vi "数据库读取.vi"(8 "error in (no error)":errorcluster caption="错误输入（无错误）", 11 "列表选择":T1(ring)) -> (0 "error out":errorcluster caption="错误输出", 1 "远程数据":string[][](table), 2 "本地数据":string[][](table), 3 "有未发送数据":bool)   [LabVIEW 2016, in "数据传输系统-03.lvlib"]
uses:
  <vilib>/Utility/sysdir.llb/System Directory Type.ctl
  <vilib>/addons/database/Connection.llb/DB Tools Open Connec (String).vi
  <vilib>/addons/database/_DB Variant To Data/Database Variant To Data.xnode
  <vilib>/addons/database/NI_Database_API.lvlib
panel:
  out "远程数据 2":string[][](table)
  out "x-y":i32[](array[numeric])
  out "大小 2":i32[](array[numeric])
  out "大小":i32[](array[numeric])
  out "待发送数据量":i32
  out "已发送数据量":i32
  out "error out 2":errorcluster caption="错误输出"
  in  "error in (no error) 2":errorcluster caption="错误输入（无错误）"
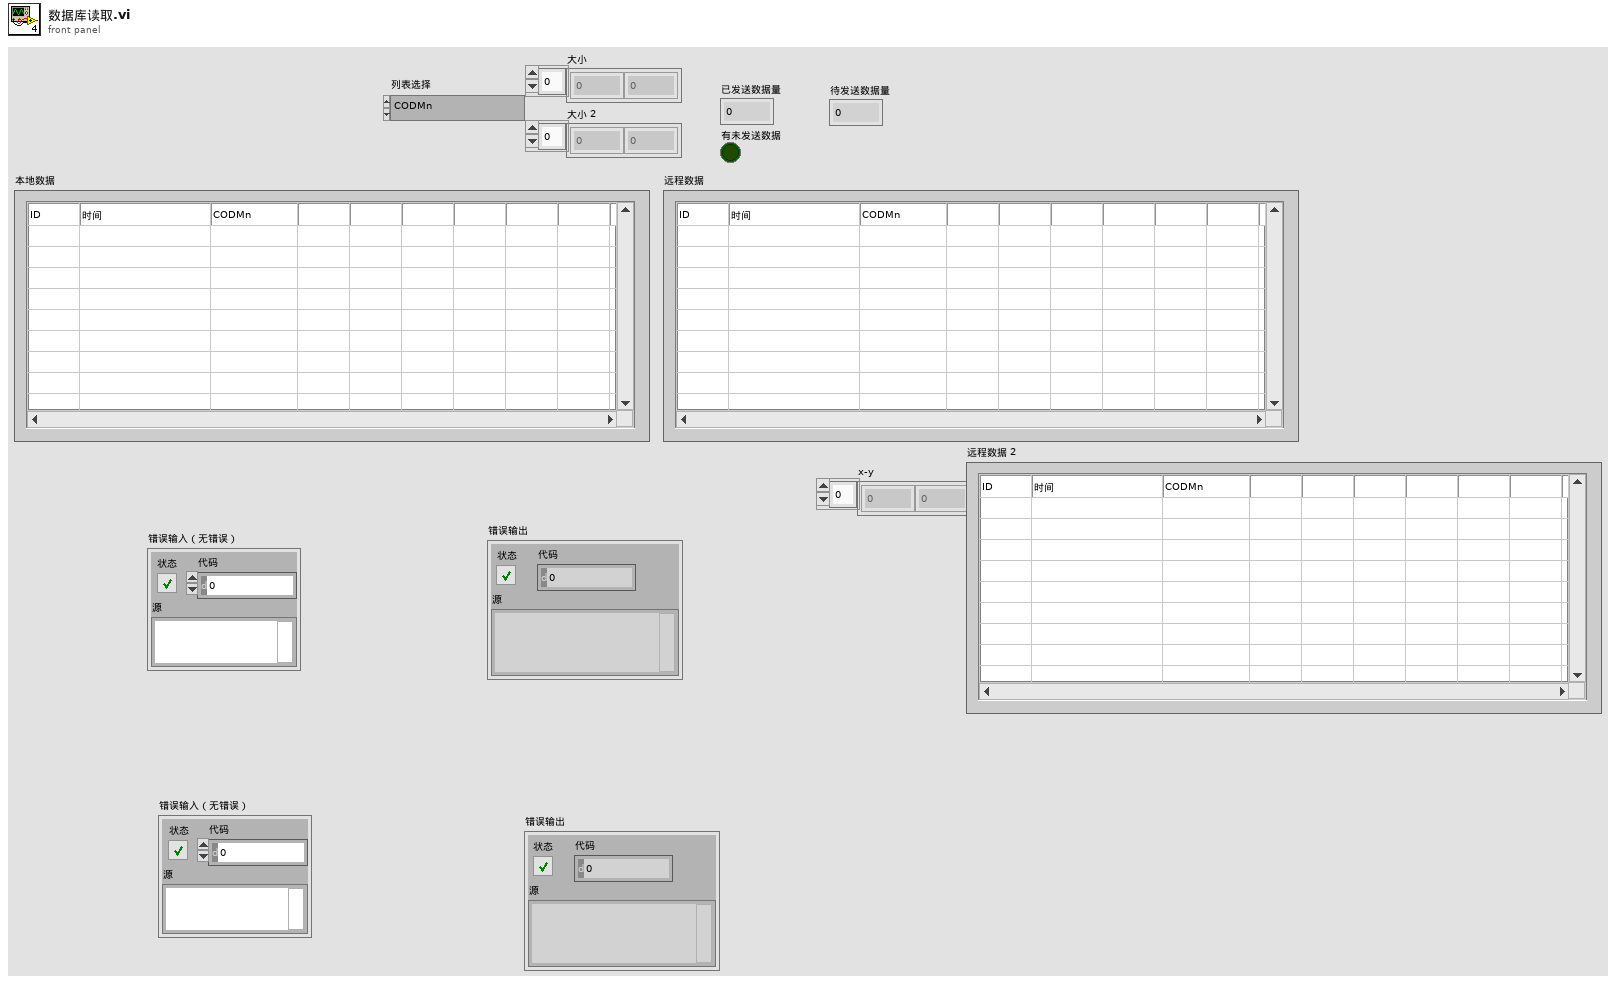
[diagram p1: front panel]
types:
  T1 = enum16{"CODMn", "CODMn空白核查", "CODMn标样核查", "氨氮", "氨氮空白核查", "氨氮标样核查", "多参数", "多参标样核查", "总磷", "总磷空白核查", "总磷标样核查", "总氮", "总氮空白核查", "总氮标样核查"}
  T2 = typedef "System Directory Type.ctl" = i32
  T3 = typedef "NI_Database_API.lvlib/Conn ObjectReference.ctl" = refnum<k1>
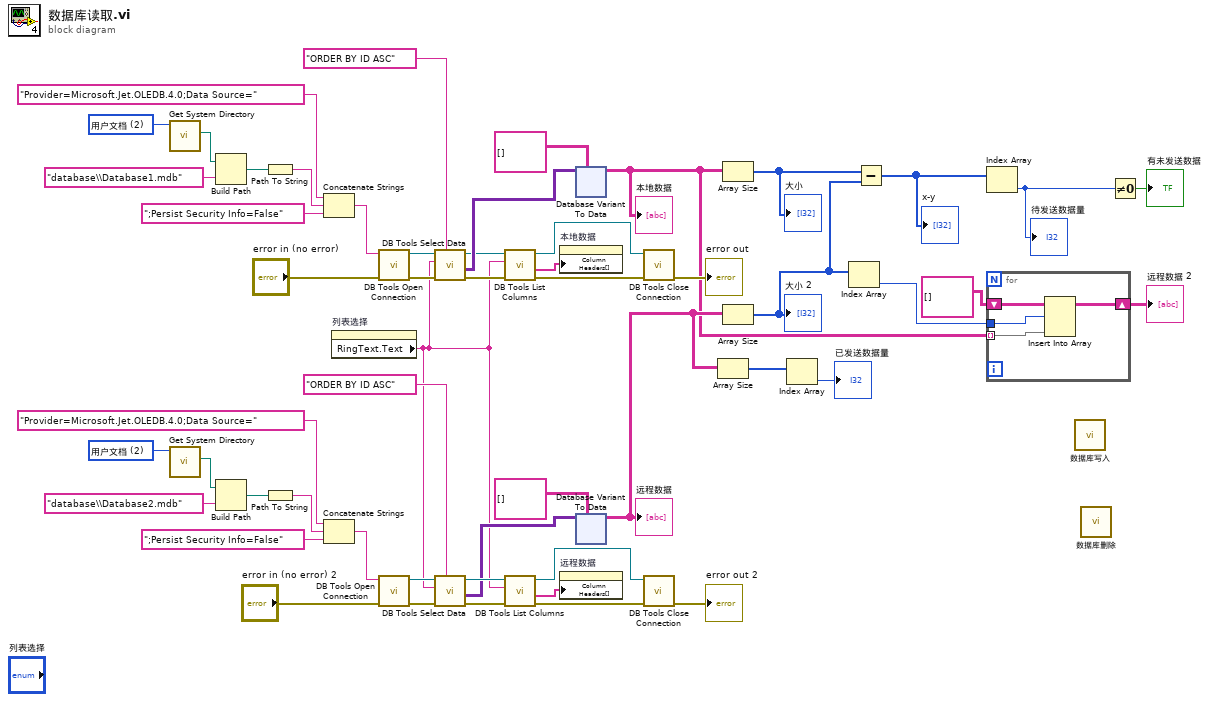
[diagram p0: block diagram]
diagram:
  w26 = T2 2 items=["用户目录"=0, "用户桌面"=1, "用户文档"=2, "用户应用程序数据"=3, "用户设置"=4, "用户临时目录"=5, "公共文档"=6, "公共应用程序数据"=7, "公共设置"=8, "公共缓存"=13, "系统核心库"=9, "系统安装库"=10, "应用程序文件"=11, "启动盘根目录"=12] ("system directory type")
  w41 = T2 2 items=["用户目录"=0, "用户桌面"=1, "用户文档"=2, "用户应用程序数据"=3, "用户设置"=4, "用户临时目录"=5, "公共文档"=6, "公共应用程序数据"=7, "公共设置"=8, "公共缓存"=13, "系统核心库"=9, "系统安装库"=10, "应用程序文件"=11, "启动盘根目录"=12] ("system directory type")
  n1 = call <vilib>:"Get System Directory.vi"("system directory type"=w41) -> ("system directory"=w39:path)  [unwired: 10 in]
  n2 = call <vilib>:"Get System Directory.vi"("system directory type"=w26) -> ("system directory"=w28:path)  [unwired: 10 in]
  n3 = Build Path(base path=w39, name or relative path="database\\Database1.mdb" ("condition")) -> (appended path=w37:path)
  n4 = Build Path(base path=w28, name or relative path="database\\Database2.mdb" ("condition")) -> (appended path=w30:path)
  n5 = Path To String(path=w37) -> (string=w36:string)
  n6 = Path To String(path=w30) -> (string=w31:string)
  n7 = Concatenate Strings("Provider=Microsoft.Jet.OLEDB.4.0;Data Source=" ("condition"), w36, ";Persist Security Info=False" ("condition")) -> (w34:string)
  n8 = Concatenate Strings("Provider=Microsoft.Jet.OLEDB.4.0;Data Source=" ("condition"), w31, ";Persist Security Info=False" ("condition")) -> (w33:string)
  n9 = property on="列表选择" class="Enum (严格)"() -> ("RingText.Text"=w11:string)  [unwired: 2 in, 2 out]
  n10 = call-poly <vilib>:"DB Tools Open Connection.vi"("error in (no error)"="error in (no error)", "connection information"=w34) -> ("error out"=w52:errorcluster, "connection reference"=w53:T3)  [unwired: 6 in]
  n11 = call-poly <vilib>:"DB Tools Open Connection.vi"("error in (no error)"="error in (no error) 2", "connection information"=w33) -> ("error out"=w21:errorcluster, "connection reference"=w20:T3)  [unwired: 6 in]
  n12 = call <vilib>:"DB Tools Select Data.vi"("condition"="ORDER BY ID ASC", "error in (no error)"=w52, "table"=w11, "connection reference"=w53) -> ("error out"=w47:errorcluster, "data"=w51:variant[][], "connection reference out"=w48:T3)  [unwired: 2 in]
  n13 = call <vilib>:"DB Tools Select Data.vi"("condition"="ORDER BY ID ASC", "error in (no error)"=w21, "table"=w11, "connection reference"=w20) -> ("error out"=w24:errorcluster, "data"=w18:variant[][], "connection reference out"=w23:T3)  [unwired: 2 in]
  n14 = call <vilib>:"DB Tools List Columns.vi"("error in (no error)"=w47, "table"=w11, "connection reference"=w48) -> ("error out"=w46:errorcluster, "columns"=w43:string[], "connection reference out"=w45:T3)  [unwired: 1 in, 1 out]
  n15 = call <vilib>:"DB Tools List Columns.vi"("error in (no error)"=w24, "table"=w11, "connection reference"=w23) -> ("error out"=w14:errorcluster, "columns"=w17:string[], "connection reference out"=w15:T3)  [unwired: 1 in, 1 out]
  n16 = property on="本地数据" class="Tbl (严格)"("Column Headers[]"=w43) -> ()  [unwired: 2 in, 2 out]
  n17 = property on="远程数据" class="Tbl (严格)"("Column Headers[]"=w17) -> ()  [unwired: 2 in, 2 out]
  n18 = xnode "Database Variant To Data"("database variant"=w51, "type"=string[][] []) -> ("data"=w3:string[][])  [unwired: 1 in, 1 out]
  "本地数据" <- w3
  n19 = xnode "Database Variant To Data"("database variant"=w18, "type"=string[][] []) -> ("data"=w10:string[][])  [unwired: 1 in, 1 out]
  "远程数据" <- w10
  n20 = call <vilib>:"DB Tools Close Connection.vi"("error in (no error)"=w46, "connection reference"=w45) -> ("error out"=→"error out":errorcluster)  [unwired: 5 in]
  n21 = call <vilib>:"DB Tools Close Connection.vi"("error in (no error)"=w14, "connection reference"=w15) -> ("error out"=→"error out 2":errorcluster)  [unwired: 5 in]
  n22 = Array Size(array=w10) -> (size(s)=w13:i32[])
  n23 = Array Size(array=w3) -> (size(s)=w6:i32[])
  "大小" <- w6
  n24 = Array Size(array=w10) -> (size(s)=w5:i32[])
  "大小 2" <- w5
  n25 = Index Array(array=w13) -> (element=→"已发送数据量":i32)  [unwired: 1 in]
  n26 = Index Array(array=w5) -> (element=w4:i32)  [unwired: 1 in]
  n27 = Subtract(x=w6, y=w5) -> (x-y=w9:i32[])
  "x-y" <- w9
  n28 = Index Array(array=w9) -> (element=w7:i32)  [unwired: 1 in]
  "待发送数据量" <- w7
  n29 = for {
    tunnel: w3 -> [w55] mode=indexing
    tunnel: w4 -> [w56]
    shift-right: [w54] -> w2
    shift-left: string[][] [] -> [w57]
    n30 = Insert Into Array(array=w57, index (row)=w56, new element=w55) -> (w54:string[][])  [unwired: 1 in]
  }
  "远程数据 2" <- w2
  n31 = call "数据库写入.vi"() -> ()  [unwired: 18 in, 2 out]
  n32 = call "数据库删除.vi"() -> ()  [unwired: 9 in, 3 out]
  n33 = Not Equal To 0?(x=w7) -> (x != 0?=→"有未发送数据":bool)
